vi "Get VI Info Data.vi"(8 "error in":errorcluster, 11 "vi reference in":refnum<vi>) -> (0 "error out":errorcluster, 2 "VI Info":cluster{"HTML":string}, 3 "vi reference out":refnum<vi>)   [LabVIEW 2019]
doc: "Get information about the VI and creates an HTML content to be used in the main viewer."
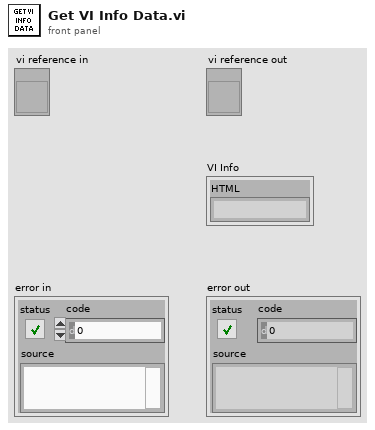
[diagram p1: front panel]
types:
  T1 = enum32{"invalid VI type", "Standard VI", "Control VI", "Global VI", "Polymorphic VI", "Configuration VI", "SubSystem", "Facade VI", "Method VI", "Statechart Diagram VI"}
  T2 = typedef "imagedata.ctl" = cluster{"image type":i32, "image depth":i32, "image":u8[], "mask":u8[], "colors":u32[], "Rectangle":cluster{"left":i16, "top":i16, "right":i16, "bottom":i16}}
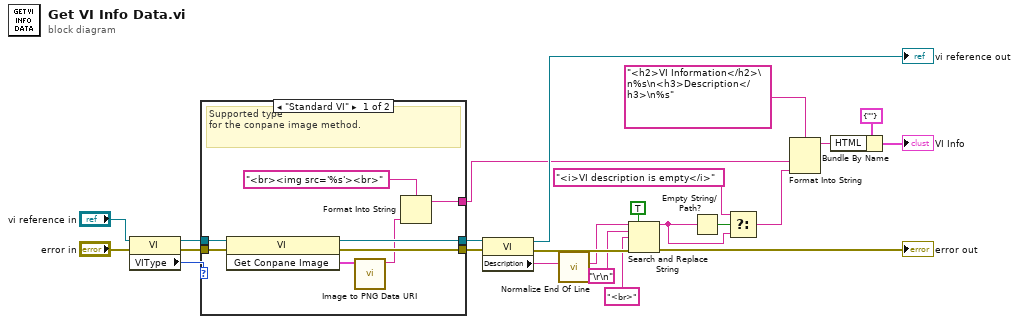
[diagram p0: block diagram]
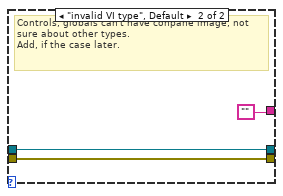
[diagram p2: hidden frame]
diagram:
  n1 = property class="VI"(reference="vi reference in", error in="error in") -> (reference out=w3:refnum<vi>, error out=w6:errorcluster, "VIType"=w4:T1)
  n2 = case shown="\"Standard VI\"" w4 {
    tunnel: w6 -> [w32 w35]
    tunnel: [w30 w35] -> w5
    tunnel: w3 -> [w31 w34]
    tunnel: [w29 w34] -> w2
    tunnel: [w25 ""] -> w1
    frame "Standard VI" {
      # "Supported type \nfor the conpane image method."
      n3 = invoke class="VI" method="Get Conpane Image"(reference=w31, error in=w32) -> (reference out=w29:refnum<vi>, error out=w30:errorcluster, "Get Conpane Image"=w28:T2)  [unwired: 1 in]
      n4 = call "Image to PNG Data URI.vi"("img data"=w28) -> ("Base64 Encoded"=w26:string)  [unwired: 9 in, 1 out]
      n5 = Format Into String(format string="<br><img src='%s'><br>" ("t"), w26) -> (resulting string=w25:string)  [unwired: 2 in, 1 out]
    }
    frame "invalid VI type", Default {
      # "Controls, globals can't have conpane image, not sure about other types. \nAdd, if the case later."
    }
  }
  n6 = property class="VI"(reference=w2, error in=w5) -> (reference out=→"vi reference out":refnum<vi>, error out=w21:errorcluster, "Description"=w22:string)
  n7 = call <vilib>:"Normalize End Of Line.vi"("string in"=w22) -> ("string out"=w19:string)  [unwired: 7 in]
  n8 = Search and Replace String(replace all?=TRUE ("replace all? (F)"), input string=w19, search string="\r\n", replace string="<br>" ("replace string (\"\")"), error in=w21) -> (result string=w11:string, error out=→"error out":errorcluster)  [unwired: 3 in, 2 out]
  n9 = Empty String/Path?(string/path=w11) -> (empty?=w12:bool)
  n10 = Select(t="<i>VI description is empty</i>", s=w12, f=w11) -> (s? t:f=w9:string)
  n11 = Format Into String(format string="<h2>VI Information</h2>\n%s\n<h3>Description</h3>\n%s", w1, w9) -> (resulting string=w13:string)  [unwired: 2 in, 1 out]
  n12 = Bundle By Name(cluster=cluster{"HTML":string} {"HTML"=""} ("VI Info"), "HTML"=w13) -> (→"VI Info":cluster{"HTML":string})
